vi "Base.Device.SetConnected.vi"(8 "error in (no error)":errorcluster, 10 "Connected?":bool, 11 "BASE.Device in":refnum<class "BASE.Device.lvclass">) -> (0 "error out":errorcluster, 3 "BASE.Device out":refnum<class "BASE.Device.lvclass">)   [LabVIEW 2019, in "BASE.Device.lvlib" / "BASE.Device.lvclass"]
uses:
  BASE.Device.lvclass
  BASE.Device.lvclass/BASE.Device.ctl
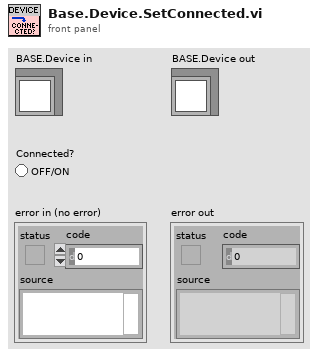
[diagram p1: front panel]
types:
  T1 = typedef "BASE.Device.lvlib/BASE.Device.lvclass/privateData--reference.ctl" = refnum<data-value>
  T2 = typedef "BASE.Device.lvlib/BASE.Device.lvclass/privateData--cluster.ctl" = cluster{"config":T3, "Connected?":bool, "Device State":variant}
  T3 = typedef "BASE.Device.lvlib/BASE.Device.lvclass/config--cluster.ctl" = cluster{"Connect Timeout":i32, "Connect Interval":u32, "Check Timeout":i32, "Check Intverval":u32, "Read Timeout":i32, "Read Interval":u32}
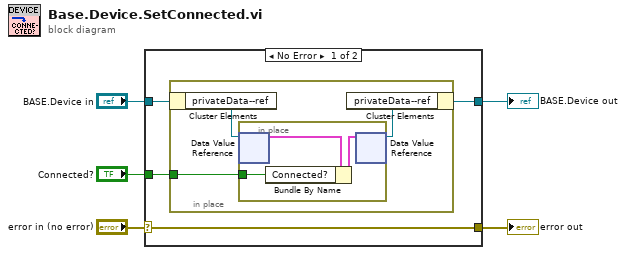
[diagram p0: block diagram]
diagram:
  n1 = case shown="No Error" "error in (no error)" {
    selector: "error in (no error)" -> [w9 w16]
    tunnel: [w9 w16] -> w1
    tunnel: [w7 w17] -> w2
    tunnel: "BASE.Device in" -> [w8 w17]
    tunnel: "Connected?" -> [w6 _]
    frame No Error {
      n2 = in-place {
        in-place-border: w6 -> [w10]
        n3 = in-place-cluster #1(w8) -> ("privateData--ref"=w12:T1)
        n4 = in-place {
          in-place-border: w10 -> [w13]
          n5 = in-place-dvr #2(w12) -> (w15:T2)  [unwired: 1 out]
          n6 = Bundle By Name(cluster=w15, "Connected?"=w13) -> (w14:T2)
          n7 = in-place-dvr #2(w14) -> (w11:T1)  [unwired: 1 out]
        }
        n8 = in-place-cluster #1("privateData--ref"=w11) -> (w7:refnum<class "BASE.Device.lvclass">)
      }
    }
    frame Error {
    }
  }
  "error out" <- w1
  "BASE.Device out" <- w2
